vi "Test_RequestInvalidTopic_ReturnError.vi"(8 "error in (no error)":errorcluster, 11 "TestCase in":refnum<class "TestTopicLookupTable.lvclass">) -> (0 "error out":errorcluster, 3 "TestCase out":refnum<class "TestTopicLookupTable.lvclass">)   [LabVIEW 2017, in "TestTopicLookupTable.lvclass"]
uses:
  TestTopicLookupTable.lvclass
  <vilib>/addons/_JKI Toolkits/VI Tester/TestCase.llb/TestCase.lvclass
  gpm_packages/@cs/mva-core/Source/Mediator/TopicLookupTable/TopicLookupTable.lvclass
  C:/Program Files (x86)/National Instruments/LabVIEW 2017/vi.lib/addons/_JKI Toolkits/VI Tester/TestCase.llb/TestCase.lvclass
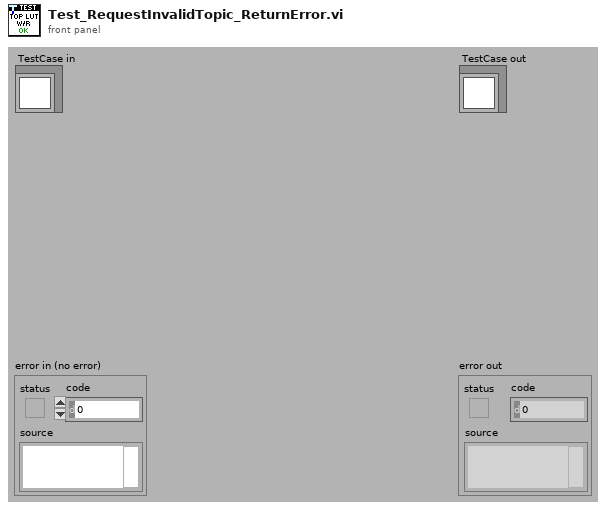
[diagram p1: front panel]
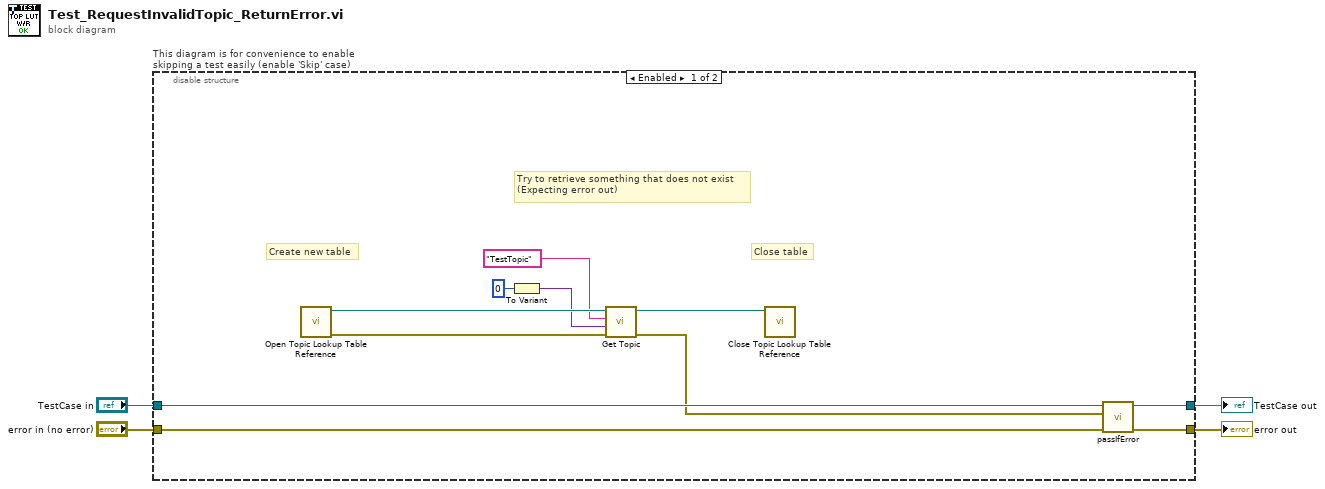
[diagram p0: block diagram]
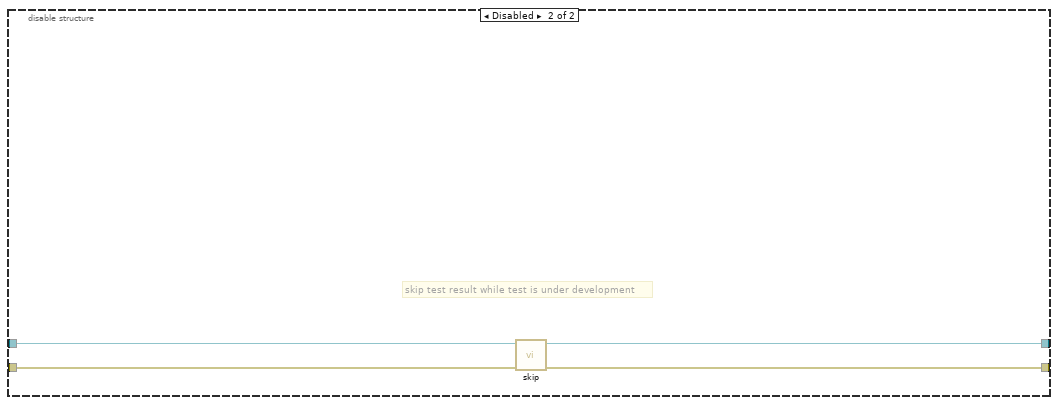
[diagram p2: hidden frame]
diagram:
  n1 = disable-structure "This diagram is for convenience to enable skipping a test easily (enable 'Skip' case)" shown="Enabled" {
    disable-tunnel: "TestCase in" -> [w15 w19]
    disable-tunnel: [w14 w17] -> w1
    disable-tunnel: [w13 w18] -> w3
    disable-tunnel: "error in (no error)" -> [w12 w16]
    frame Enabled {
      # "Close table"
      # "Create new table"
      # "Try to retrieve something that does not exist\n(Expecting error out)"
      n2 = call "Open Topic Lookup Table Reference.vi"() -> ("error out"=w10:errorcluster, "TopicLookupTable Reference"=w11:refnum<data-value>)  [unwired: 10 in]
      n3 = To Variant(anything=0) -> (Variant=w5:variant)
      n4 = call "Get Topic.vi"("error in (no error)"=w10, "Topic Type"=w5, "Topic Name"="TestTopic", "TopicLookupTable"=w11) -> ("error out"=w7:errorcluster, "TopicLookupTable"=w9:refnum<data-value>)  [unwired: 5 in, 1 out]
      n5 = call "Close Topic Lookup Table Reference.vi"("TopicLookupTable"=w9) -> ()  [unwired: 10 in, 1 out]
      n6 = call-dynamic "passIfError.vi"("error in (no error)"=w12, "error"=w7, "TestCase in"=w15) -> ("error out"=w13:errorcluster, "TestCase out"=w14:refnum<class "TestTopicLookupTable.lvclass">)  [unwired: 7 in]
    }
    frame Disabled {
      # "skip test result while test is under development"
      n7 = call <vilib>:"skip.vi"("error in (no error)"=w16, "TestCase in"=w19) -> ("error out"=w18:errorcluster, "TestCase out"=w17:refnum<class "TestTopicLookupTable.lvclass">)  [unwired: 8 in]
    }
  }
  "error out" <- w3
  "TestCase out" <- w1
